vi "Reset USB&temp v 1 test.vi"(7 "Test":bool=TRUE) -> (0 "Reset Error":bool)   [LabVIEW 2017]
uses:
  <vilib>/Platform/TimedLoop/XDataNode/timing_clust.ctl
  <vilib>/Platform/TimedLoop/XDataNode/nitl_modes.ctl
  <vilib>/Platform/TimedLoop/XDataNode/wakeup.ctl
  <vilib>/platform/TimedLoop/XDataNode/XDataNode.xnode
  <vilib>/Platform/TimedLoop/XDataNode/XDNodeRunTimeDep.lvlib
panel:
  out "Reset Time Out":dbl
  out "Message":string
  in  "End Reset Routine":bool
  # "RESET USB $ TEMP"
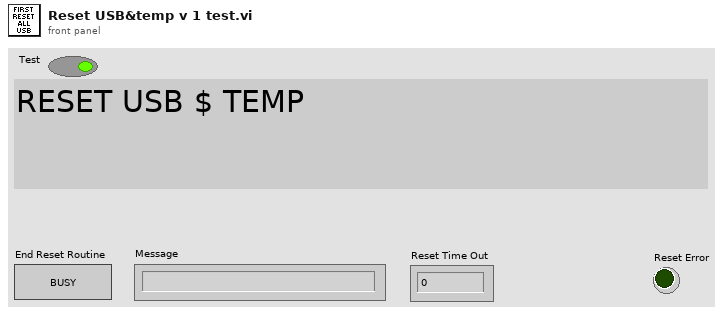
[diagram p1: front panel]
types:
  T1 = typedef "XDNodeRunTimeDep.lvlib/timing_clust.ctl" = cluster{"Expected End [f-1]":u64, "Actual End [f-1]":u64, "Finished Late? [f-1]":bool, "Expected End [i-1]":u64, "Actual End [i-1]":u64, "Finished Late? [i-1]":bool, "Expected Start [i]":u64, "Actual Start [i]":u64, "Expected Start [f]":u64, "Actual Start [f]":u64, "Source Name":string, "Structure Name":string, "Period":i64, "Deadline":i64, "Offset":i64, "Start":i64, "Priority":i32, "Timeout":i32, "Mode":T2, "Wakeup Reason":T3, "Error":errorcluster, "Source Type":string, "Secondary Source Type":string, "Global End Time":u64, "Global Start Time":u64, "Frame Duration":u64, "Iteration Duration":u64, "Assigned CPU":i32, "I/O Scan Engine Mode":u32}
  T2 = typedef "XDNodeRunTimeDep.lvlib/nitl_modes.ctl" = enum32{"No Change", "Process missed periods, maintain original phase", "Discard missed periods, maintain original phase", "Process missed periods, ignore original phase", "Discard missed periods, ignore original phase"}
  T3 = typedef "XDNodeRunTimeDep.lvlib/wakeup.ctl" = enum32{"Normal", "Aborted", "Asynchronous wakeup", "Timing source error", "Timed loop error", "Timeout"}
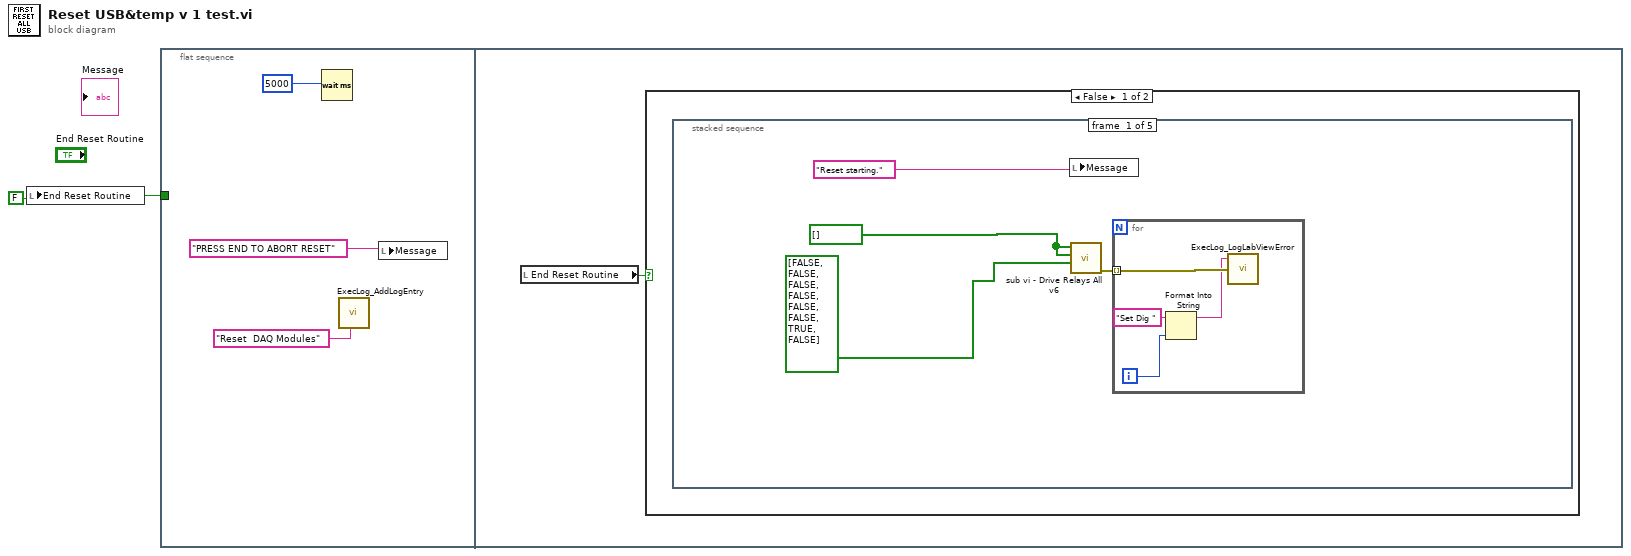
[diagram p0: block diagram]
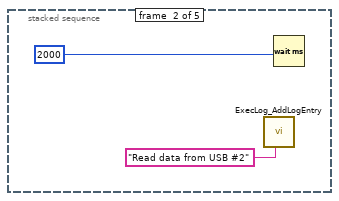
[diagram p2: hidden frame]
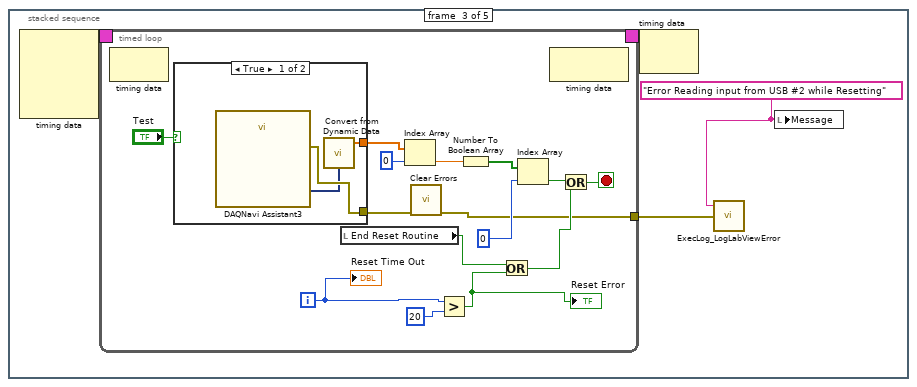
[diagram p3: hidden frame]
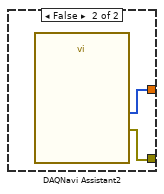
[diagram p4: hidden frame]
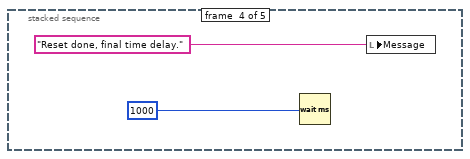
[diagram p5: hidden frame]
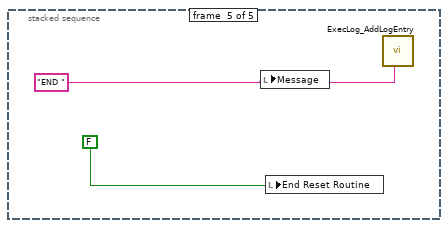
[diagram p6: hidden frame]
diagram:
  w1 = FALSE
  n1 = local write "End Reset Routine"(w1) -> ()
  n2 = flat-sequence {
    tunnel: w1 -> [_]
    frame #0 {
      n3 = Wait (ms)(milliseconds to wait=5000) -> ()  [unwired: 1 out]
      n4 = call "ExecLog_AddLogEntry.vi"("Msg"="Reset  DAQ Modules") -> ()  [unwired: 7 in, 3 out]
      n5 = local write "Message"("PRESS END TO ABORT RESET") -> ()
    }
    frame #1 {
      n6 = local read "End Reset Routine"() -> (w5:bool)
      n7 = case shown="False" w5 {
        frame False {
          n8 = stacked-sequence {
            frame #0 {
              w8 = bool[] []
              n9 = local write "Message"("Reset starting.") -> ()
              n10 = call "sub vi - Drive Relays All v6.vi"("Array #2"=bool[] [FALSE, FALSE, FALSE, FALSE, FALSE, FALSE, TRUE, FALSE], "Array #1"=w8, "Array #0"=w8) -> ("error Array"=w6:errorcluster[])  [unwired: 8 in]
              n11 = for {
                tunnel: w6 -> [w13] mode=indexing
                i -> [w11]
                n12 = Format Into String(initial string="Set Dig ", w11) -> (resulting string=w10:string)  [unwired: 2 in, 1 out]
                n13 = call "ExecLog_LogLabViewError.vi"("error IO"=w13, "string 1"=w10) -> ()  [unwired: 2 in, 1 out]
              }
            }
            frame #1 {
              n14 = call "ExecLog_AddLogEntry.vi"("Msg"="Read data from USB #2") -> ()  [unwired: 7 in, 3 out]
              n15 = Wait (ms)(milliseconds to wait=2000) -> ()  [unwired: 1 out]
            }
            frame #2 {
              w16 = "Error Reading input from USB #2 while Resetting"
              n16 = node-c288() -> (w19:T1)  [unwired: 4 in]
              n17 = timed-loop {
                timing: w19 -> [_]
                timing-out: [_] -> w18
                tunnel: [w20] -> w17
                i -> [w22]
                stop <- w30 stop-if-true
                n18 = node-c288() -> ()  [unwired: 1 in, 1 out]
                n19 = case shown="True" "Test" {
                  tunnel: [w35 w39] -> w28
                  tunnel: [w37 w38] -> w27
                  frame True {
                    n20 = call "DAQNavi Assistant3"() -> ("error out"=w37:errorcluster, "data out(DDT)"=w36:dynamicdata)  [unwired: 26 in]
                    n21 = call "Convert from Dynamic Data"("Dynamic Data Type"=w36) -> ("Array"=w35:dbl[])  [unwired: 3 in]
                  }
                  frame False {
                    n22 = call "DAQNavi Assistant2"() -> ("error out"=w38:errorcluster, "dataOut(U8Array)"=w39:u8[])  [unwired: 26 in]
                  }
                }
                n23 = local read "End Reset Routine"() -> (w26:bool)
                n24 = Index Array(array=w28, index=0) -> (element=w32:dbl)
                n25 = call <vilib>:"Clear Errors.vi"("error in (no error)"=w27) -> ("error out"=w20:errorcluster)  [unwired: 5 in, 1 out]
                n26 = Greater?(x=w22, y=20) -> (0:w23:bool)
                "Reset Error" <- w23
                n27 = Number To Boolean Array(number=w32) -> (Boolean array=w33:bool[])
                n28 = Or(x=w26, y=w23) -> (x .or. y?=w24:bool)
                n29 = Index Array(array=w33, index=0) -> (element=w29:bool)
                n30 = node-c288() -> ()  [unwired: 1 in, 1 out]
                n31 = Or(x=w29, y=w24) -> (x .or. y?=w30:bool)
                "Reset Time Out" <- w22
              }
              n32 = node-c288(w18) -> ()  [unwired: 1 out]
              n33 = call "ExecLog_LogLabViewError.vi"("error IO"=w17, "string 1"=w16) -> ()  [unwired: 2 in, 1 out]
              n34 = local write "Message"(w16) -> ()
            }
            frame #3 {
              n35 = Wait (ms)(milliseconds to wait=1000) -> ()  [unwired: 1 out]
              n36 = local write "Message"("Reset done, final time delay.") -> ()
            }
            frame #4 {
              w46 = "END "
              n37 = local write "Message"(w46) -> ()
              n38 = local write "End Reset Routine"(FALSE) -> ()
              n39 = call "ExecLog_AddLogEntry.vi"("Msg"=w46) -> ()  [unwired: 7 in, 3 out]
            }
          }
        }
        frame True {
        }
      }
    }
  }
